vi "jsonStructureInfo.vi"(8 "error in (no error)":errorcluster, 10 "path":string, 11 "d in":i64) -> (0 "error out":errorcluster, 1 "value out":i64, 2 "count":i32, 3 "d out":i64)   [LabVIEW 2015, in "rapidjson wrapper.lvlib"]
uses:
  rapidjson wrapper.lvlib
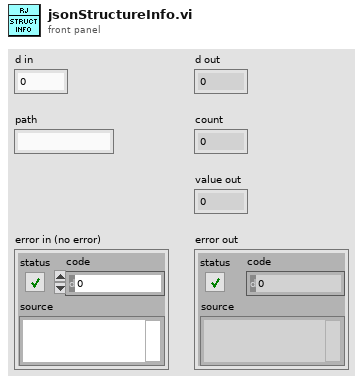
[diagram p1: front panel]
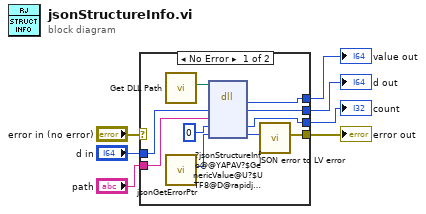
[diagram p0: block diagram]
diagram:
  n1 = case shown="No Error" "error in (no error)" {
    selector: "error in (no error)" -> [_ w19]
    tunnel: [w14 w19] -> w7
    tunnel: "d in" -> [w13 w18]
    tunnel: [w12 w18] -> w4
    tunnel: "path" -> [w11 _]
    tunnel: [w10 _] -> w2
    tunnel: [w9 _] -> w1
    frame No Error {
      n2 = call "Get DLL Path.vi"() -> ("Path"=w17:path)  [unwired: 11 in]
      n3 = call "jsonGetErrorPtr.vi"() -> ("return type"=w16:i64)  [unwired: 10 in, 1 out]
      n4 = dll-call lib="C:/Users/tblair/Documents/Git Projects/rapidjson-for-LabVIEW/lvrjs/Debug/lvrjs.dll" fn="?jsonStructureInfo@@YAPAV?$GenericValue@U?$UTF8@D@rapidjson@@V?$MemoryPoolAllocator@VCrtAllocator@rapidjson@@@2@@rapidjson@@PAV?$GenericDocument@U?$UTF8@D@rapidjson@@V?$MemoryPoolAllocator@VCrtAllocator@rapidjson@@@2@VCrtAllocator@2@@2@PADAAH0@Z"(path in=w17, "d"=w13, "path"=w11, "count"=0, "jsonError"=w16) -> ("return type"=w10:i64, "d"=w12:i64, "count"=w9:i32, "jsonError"=w15:i64)  [unwired: 3 in, 2 out]
      n5 = call "JSON error to LV error.vi"("jsonError"=w15) -> ("error out"=w14:errorcluster)  [unwired: 10 in]
    }
    frame Error {
    }
  }
  "error out" <- w7
  "d out" <- w4
  "value out" <- w2
  "count" <- w1
